vi "Get Waveform.vi"(8 "error in (no error)":errorcluster, 10 "Save data":bool, 11 "Tektronix Driver in":refnum<class "Tektronix 7000 Driver.lvclass">) -> (0 "error out":errorcluster, 2 "Waveform":waveform(dbl), 3 "Tektronix Driver out":refnum<class "Tektronix 7000 Driver.lvclass">)   [LabVIEW 2020, in "Tektronix 7000 Driver.lvclass"]
uses:
  Tektronix 7000 Driver.lvclass
  C:/GitHub/NHMFL_Core/Libraries/Instruments/Tektronix/Tektronix Driver/Tektronix Driver.lvclass
  <instrlib>/Tektronix 7000 Series/Tektronix 7000 Series.lvlib
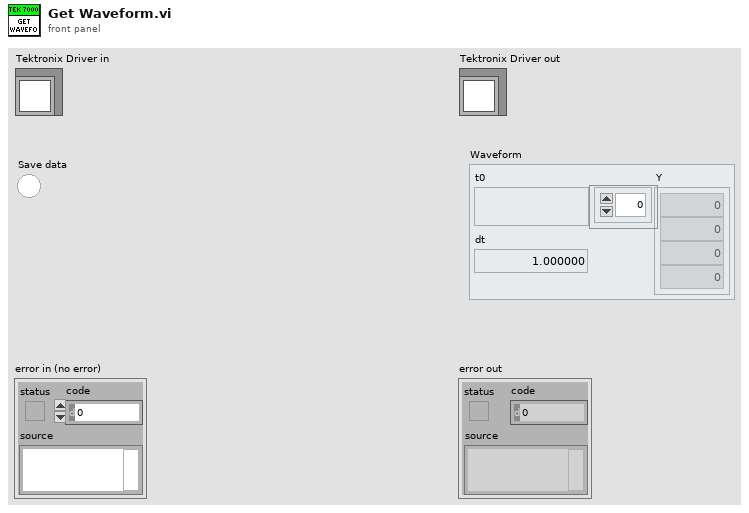
[diagram p1: front panel]
types:
  T1 = typedef "Tektronix Configuration.ctl" = cluster{"Channel":i32, "Number of averages":i32, "Input impedace":enum16{"1 M Ohm", "50 Ohm"}, "Vertical coupling":enum16{"AC", "DC", "Ground"}}
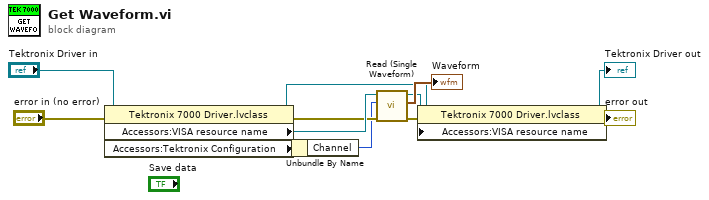
[diagram p0: block diagram]
diagram:
  n1 = property class="Tektronix 7000 Driver.lvclass"(reference="Tektronix Driver in", error in="error in (no error)") -> (reference out=w2:refnum<class "Tektronix 7000 Driver.lvclass">, error out=w11:errorcluster, "Accessors:VISA resource name"=w12:refnum<visa-resource-name>, "Accessors:Tektronix Configuration"=w9:T1)
  n2 = Unbundle By Name(w9) -> ("Channel"=w10:i32)
  n3 = call <instrlib>:"Read (Single Waveform).vi"("error in (no error)"=w11, "Channel (0: Channel 1)"=w10, "VISA resource name"=w12) -> ("error out"=w6:errorcluster, "Waveform Data"=→"Waveform":waveform(dbl), "VISA resource name out"=w7:refnum<visa-resource-name>)  [unwired: 6 in]
  n4 = property class="Tektronix 7000 Driver.lvclass"(reference=w2, error in=w6, "Accessors:VISA resource name"=w7) -> (reference out=→"Tektronix Driver out":refnum<class "Tektronix 7000 Driver.lvclass">, error out=→"error out":errorcluster)
